vi "FGV Event.vi"(8 "error in (no error)":errorcluster, 10 "FGV Event State":T1, 11 "user event in":refnum<user-event>) -> (0 "error out":errorcluster, 3 "user event out":refnum<user-event>)   [LabVIEW 2023, in "Controller.lvlib"]
uses:
  Controller.lvlib
  Events/Controls/FGV Event State.ctl
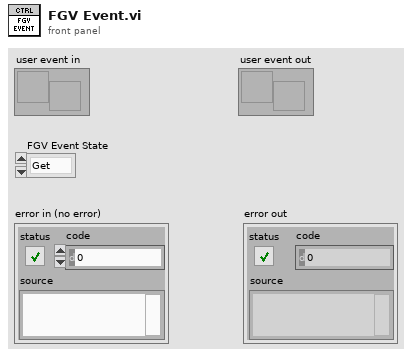
[diagram p1: front panel]
types:
  T1 = typedef "FGV Event State.ctl" = enum16{"Get", "Set"}
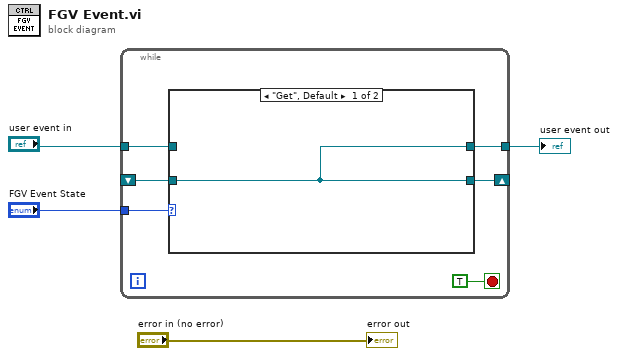
[diagram p0: block diagram]
diagram:
  n1 = while {
    tunnel: "FGV Event State" -> [w9]
    tunnel: [w8] -> w2
    tunnel: "user event in" -> [w7]
    shift-right: [w6] -> _
    shift-left: _ -> [w5]
    stop <- TRUE stop-if-true
    n2 = case shown="\"Get\", Default" w9 {
      tunnel: [w11 w12] -> w8
      tunnel: w7 -> [_ w12]
      tunnel: [w11 w12] -> w6
      tunnel: w5 -> [w11 _]
      frame "Get", Default {
      }
      frame "Set" {
      }
    }
  }
  "user event out" <- w2
  "error out" <- "error in (no error)"
